vi "verify_SN_format_new.vi"(8 "error in (no error)":errorcluster, 10 "rules list":string[][](array[string]), 11 "SN in":string) -> (0 "error out":errorcluster, 1 "SN status":enum16{"SN PASS", "SN FAIL"}(ring), 2 "message":string, 3 "SN out":string)   [LabVIEW 2024]
uses:
  Type Definitions/verify_SN_format_states.ctl
  Type Definitions/verify_SN_format_control.ctl
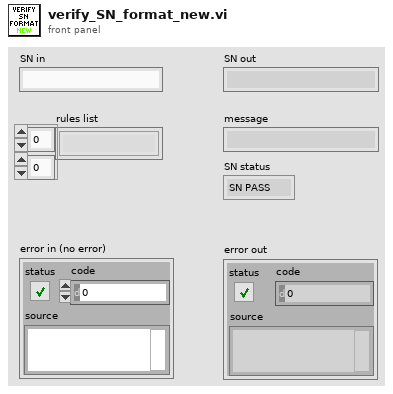
[diagram p1: front panel]
types:
  T1 = typedef "verify_SN_format_control.ctl" = cluster{"Message":string, "Product Name":string[], "Reg. Expresion":string[], "match?":bool, "SN out":string, "SN status":enum16{"SN PASS", "SN FAIL"}}
  T2 = typedef "verify_SN_format_states.ctl" = enum16{"Initialize", "Get Product Names & RegExs", "Check Empty RegExp.", "Check SN agst. RegExps.", "Error", "Shutdown"}
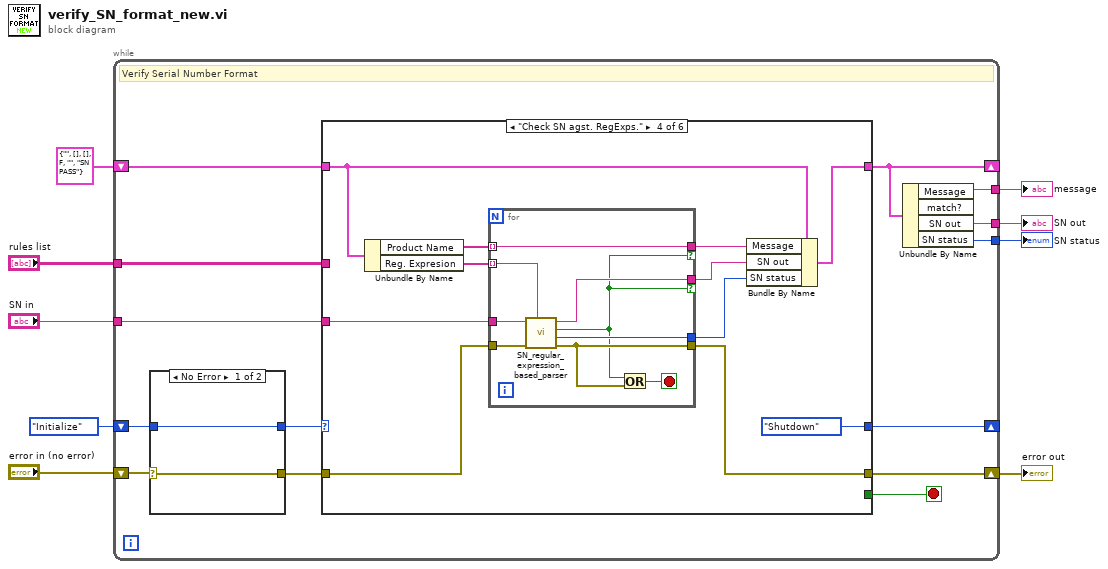
[diagram p0: block diagram]
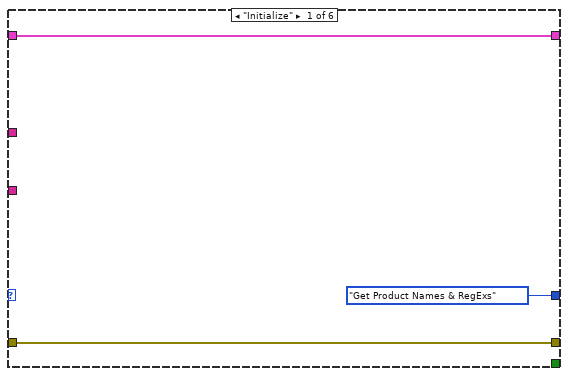
[diagram p2: hidden frame]
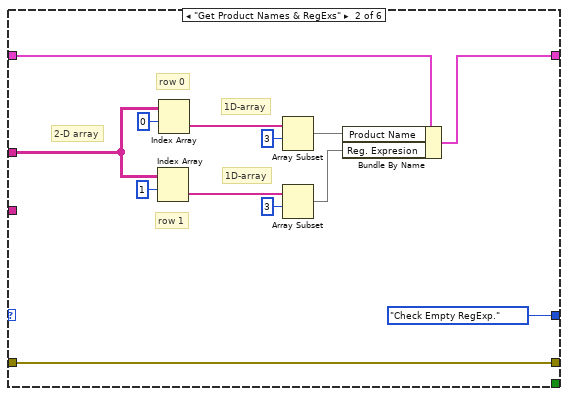
[diagram p3: hidden frame]
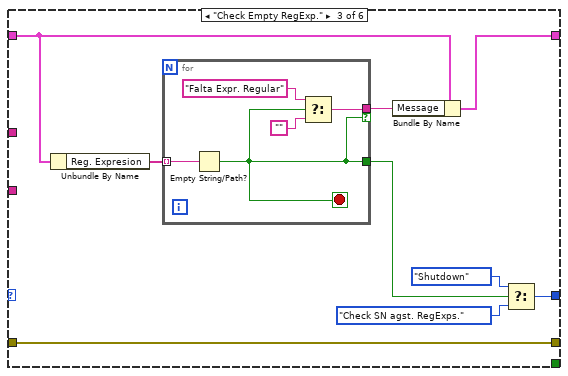
[diagram p4: hidden frame]
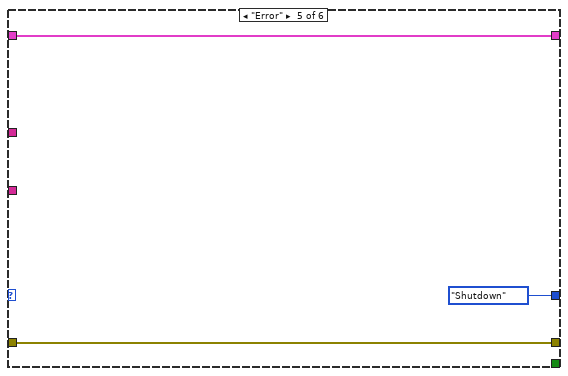
[diagram p5: hidden frame]
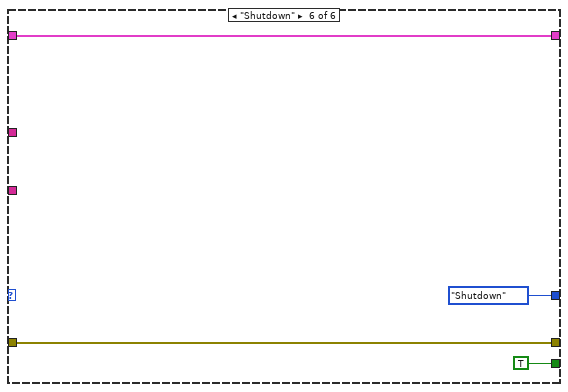
[diagram p6: hidden frame]
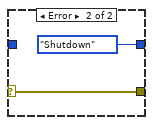
[diagram p7: hidden frame]
diagram:
  n1 = while {
    shift-right: [w19] -> w7
    shift-left: "error in (no error)" -> [w23]
    shift-right: [w14] -> _
    shift-left: T1 {"Message"="", "Product Name"=[], "Reg. Expresion"=[], "match?"=FALSE, "SN out"="", "SN status"=enum."SN PASS"} -> [w18]
    shift-right: [w17] -> _
    shift-left: verify_SN_format_states."Initialize" -> [w21]
    tunnel: "rules list" -> [w16]
    tunnel: [w13] -> w4
    tunnel: "SN in" -> [w12]
    tunnel: [w11] -> w2
    tunnel: [w10] -> w1
    stop <- w15 stop-if-true
    # "Verify Serial Number Format"
    n2 = case shown="No Error" w23 {
      selector: w23 -> [w82 w83]
      tunnel: [w82 w83] -> w22
      tunnel: w21 -> [w81 _]
      tunnel: [w81 verify_SN_format_states."Shutdown"] -> w20
      frame No Error {
      }
      frame Error {
      }
    }
    n3 = case shown="\"Check SN agst. RegExps.\"" w20 {
      tunnel: w22 -> [w26 w39 w48 w64 w76 w80]
      tunnel: [w26 w39 w48 w63 w76 w80] -> w19
      tunnel: w18 -> [w25 w38 w46 w62 w75 w79]
      tunnel: [w25 w37 w45 w59 w75 w79] -> w14
      tunnel: [verify_SN_format_states."Get Product Names & RegExs" verify_SN_format_states."Check Empty RegExp." w43 verify_SN_format_states."Shutdown" ("t") verify_SN_format_states."Shutdown" ("t") verify_SN_format_states."Shutdown" ("t")] -> w17
      tunnel: w16 -> [_ w33 _ _ _ _]
      tunnel: [_ _ _ _ _ TRUE] -> w15
      tunnel: w12 -> [_ _ _ w60 _ _]
      frame "Initialize" {
      }
      frame "Get Product Names & RegExs" {
        # "1D-array"
        # "1D-array"
        # "2-D array"
        # "row 1"
        # "row 0"
        n4 = Index Array "Index Array"(array=w33, index (row)=1) -> (element=w29:string[])  [unwired: 1 in]
        n5 = Index Array(array=w33, index (row)=0) -> (element=w30:string[])  [unwired: 1 in]
        n6 = Array Subset "Array Subset"(array=w30, index=3) -> (w28:string[])  [unwired: 1 in]
        n7 = Array Subset(array=w29, index=3) -> (w27:string[])  [unwired: 1 in]
        n8 = Bundle By Name(cluster=w38, "Product Name"=w28, "Reg. Expresion"=w27) -> (w37:T1)
      }
      frame "Check Empty RegExp." {
        n9 = Unbundle By Name(w46) -> ("Reg. Expresion"=w47:string[])
        n10 = for {
          tunnel: w47 -> [w53] mode=indexing
          tunnel: [w51] -> w44 if=w49
          tunnel: [w49] -> w42
          stop <- w49 stop-if-true
          n11 = Empty String/Path?(string/path=w53) -> (empty?=w49:bool)
          n12 = Select(t="Falta Expr. Regular", s=w49, f="") -> (s? t:f=w51:string)
        }
        n13 = Bundle By Name(cluster=w46, "Message"=w44) -> (w45:T1)
        n14 = Select(t=verify_SN_format_states."Shutdown", s=w42, f=verify_SN_format_states."Check SN agst. RegExps." ("t")) -> (s? t:f=w43:T2)
      }
      frame "Check SN agst. RegExps." {
        n15 = Unbundle By Name(w62) -> ("Product Name"=w61:string[], "Reg. Expresion"=w55:string[])
        n16 = for {
          tunnel: w61 -> [w68] mode=indexing
          tunnel: w64 -> [w73]
          tunnel: [w71] -> w63
          tunnel: [w69] -> w57 if=w65
          tunnel: [w68] -> w58 if=w65
          tunnel: w60 -> [w70]
          tunnel: w55 -> [w67] mode=indexing
          tunnel: [w66] -> w54
          stop <- w72 stop-if-true
          n17 = call "SN_regular_expression_based_parser.vi"("regular expression"=w67, "error in (no error)"=w73, "SN in"=w70) -> ("error out"=w71:errorcluster, "SN status"=w66:enum16{"SN PASS", "SN FAIL"}, "match?"=w65:bool, "SN out"=w69:string)  [unwired: 5 in]
          n18 = Or(x=w65, y=w71) -> (x .or. y?=w72:bool)
        }
        n19 = Bundle By Name(cluster=w62, "Message"=w58, "SN out"=w57, "SN status"=w54) -> (w59:T1)
      }
      frame "Error" {
      }
      frame "Shutdown" {
      }
    }
    n20 = Unbundle By Name(w14) -> ("Message"=w13:string, "SN out"=w11:string, "SN status"=w10:enum16{"SN PASS", "SN FAIL"})  [unwired: 1 out]
  }
  "message" <- w4
  "SN out" <- w2
  "error out" <- w7
  "SN status" <- w1
